vi "Add New Channel.vi"(0 "Node Ptr":T1 format="%.0x") -> ()   [LabVIEW 2023, in "Embedded TDMS Logger System Explorer.lvlib"]
uses:
  Embedded TDMS Logger System Explorer.lvlib
  <vilib>/NI VeriStand/Custom Device API/Custom Device Item Ref.ctl
  Shared/Meta Data Item.ctl
  <vilib>/NI VeriStand/Custom Device API/Custom Device Channel.ctl
  <vilib>/NI VeriStand/Custom Device API/Custom Device Channel Type.ctl
  Shared/Constants.vi
  <vilib>/NI VeriStand/Custom Device API/Set Item Property (Boolean).vi
  <vilib>/NI VeriStand/Custom Device API/Set Item Property (Variant).vi
  Shared/Embedded TDMS Logger Shared.lvlib
  <vilib>/NI VeriStand/Custom Device API/Custom Device API.lvlib
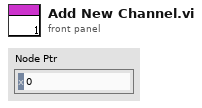
[diagram p1: front panel]
types:
  T1 = typedef "Custom Device API.lvlib/Custom Device Item Ref.ctl" = u64
  T2 = typedef "Custom Device API.lvlib/Custom Device Channel.ctl" = cluster{"Type":T3, "Units":string, "Default Value":dbl, "Faultable":bool, "Scalable":bool}
  T3 = typedef "Custom Device API.lvlib/Custom Device Channel Type.ctl" = enum16{"Input", "Output"}
  T4 = typedef "Embedded TDMS Logger Shared.lvlib/Meta Data Item.ctl" = cluster{"Key":string, "Value":string}
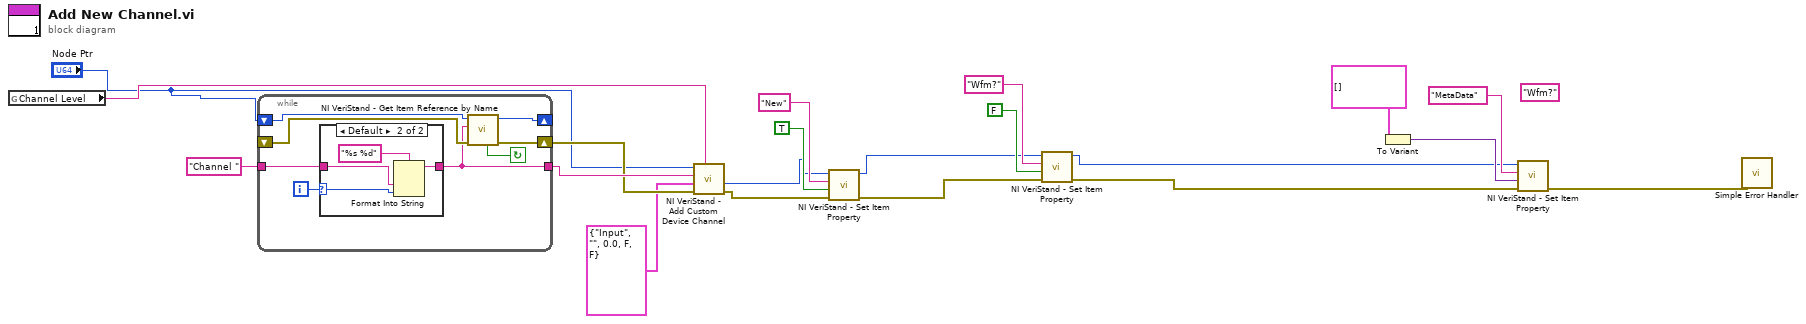
[diagram p0: block diagram]
diagram:
  (unwired) "Wfm?" ("Property Name")
  n1 = global read "Constants.vi" "Channel Level"() -> (w14:string)
  n2 = while {
    shift-right: [w22] -> w16
    shift-left: _ -> [w26]
    shift-right: [w24] -> _
    shift-left: "Node Ptr" -> [w25]
    tunnel: "Channel " ("group name") -> [w27]
    tunnel: [w21] -> w17
    i -> [w28]
    stop <- w23 continue-if-true
    n3 = case shown="Default" w28 {
      selector: w28 -> [_ w31]
      tunnel: w27 -> [w29 w32]
      tunnel: [w29 w30] -> w21
      frame 0 {
      }
      frame Default {
        n4 = Format Into String(format string="%s %d", w32, w31) -> (resulting string=w30:string)  [unwired: 2 in, 1 out]
      }
    }
    n5 = call <vilib>:"NI VeriStand - Get Item Reference by Name.vi"("error in (no error)"=w26, "Item Name"=w21, "Parent Ref in"=w25) -> ("error out"=w22:errorcluster, "Parent Ref out"=w24:T1, "Found"=w23:bool)  [unwired: 6 out]
  }
  n6 = call <vilib>:"NI VeriStand - Add Custom Device Channel.vi"("GUID (Default Channel)"=w14, "error in (no error)"=w16, "Channel"=T2 {"Type"=enum."Input", "Units"="", "Default Value"=0.0, "Faultable"=FALSE, "Scalable"=FALSE}, "Channel Name"=w17, "Parent Ref in"="Node Ptr") -> ("error out"=w15:errorcluster, "Channel Ref"=w13:T1)  [unwired: 3 in, 2 out]
  n7 = call-poly <vilib>:"NI VeriStand - Set Item Property.vi"("error in (no error)"=w15, "Value"=TRUE, "Property Name"="New", "Item Ref in"=w13) -> ("error out"=w9:errorcluster, "Item Ref out"=w10:T1)  [unwired: 5 in, 1 out]
  n8 = call-poly <vilib>:"NI VeriStand - Set Item Property.vi"("error in (no error)"=w9, "Value"=FALSE, "Property Name"="Wfm?", "Item Ref in"=w10) -> ("error out"=w1:errorcluster, "Item Ref out"=w2:T1)  [unwired: 5 in, 1 out]
  n9 = To Variant(anything=T4[] []) -> (Variant=w7:variant)
  n10 = call-poly <vilib>:"NI VeriStand - Set Item Property.vi"("error in (no error)"=w1, "Value"=w7, "Property Name"="MetaData", "Item Ref in"=w2) -> ("error out"=w5:errorcluster)  [unwired: 5 in, 2 out]
  n11 = call <vilib>:"Simple Error Handler.vi"("error in (no error)"=w5) -> ()  [unwired: 4 in, 5 out]
